vi "Final Project.vi"() -> ()   [LabVIEW 2019]
uses:
  <vilib>/vision/Pattern Matching.llb/IMAQ GM Match Report.ctl
  Control 1.ctl
  <vilib>/MakerHub/LINX/Public/Peripherals/PWM/PWM Set Duty Cycle 1 Chan.vi
  <vilib>/MakerHub/LINX/Public/Peripherals/Digital/Digital Write N Chans.vi
  <vilib>/MakerHub/LINX/Private/Local IO/LinxDigitalWrite.vi
  <vilib>/MakerHub/LINX/Public/Utilities/Check Channel.vi
  <vilib>/MakerHub/LINX/Public/Utilities/Open Serial.vi
  <vilib>/Instr/_visa.llb/VISA Configure Serial Port (Instr).vi
  <vilib>/MakerHub/LINX/Public/Peripherals/PWM/PWM Set Duty Cycle N Chans.vi
  <vilib>/MakerHub/LINX/Private/Utilties/Generate Error.vi
  <vilib>/MakerHub/LINX/LMH-LINX.lvlib
panel:
  in  "Error In":errorcluster
  out "STATE":T1
  out "concatenated string 20":string
  out "concatenated string 19":string
  out "concatenated string 18":string
  out "concatenated string 17":string
  out "concatenated string 16":string
  out "concatenated string 15":string
  out "concatenated string 14":string
  out "concatenated string 13":string
  out "concatenated string 12":string
  out "concatenated string 11":string
  out "concatenated string 10":string
  out "concatenated string 9":string
  out "concatenated string 8":string
  out "concatenated string 7":string
  out "concatenated string 6":string
  out "concatenated string 5":string
  out "concatenated string 4":string
  out "concatenated string 3":string
  out "concatenated string 2":string
  out "concatenated string":string
  out "Calibrated Matches (Pattern Matching 1)":T2[](array[typedef]) {"Correlation Score" format="%.2f"; "Target Template Curve Score" format="%.2f"; "Template Target Curve Score" format="%.2f"; "Bounding Box"."y" format="%.2f"; "Bounding Box"."x" format="%.2f"; "Position"."y" format="%.2f"; "Position"."x" format="%.2f"; "Score" format="%.2f"; "Scale" format="%.2f"; "Angle" format="%.2f"; "Occlusion %" format="%.2f"}
  out "Tab Control":T3(tab)
  in  "Start":bool
  in  "Serial Port":refnum<visa-resource-name>="N/A"
  in  "Duty Cycle (0-1)":dbl(slide) min=0.0 max=1.0 step=5e-05 scale=0.0..1.0
  in  "Values":bool[](array[boolean])
  in  "Start Image Processing":bool
  in  "STOP BUTTON":bool
  in  "OK Button":bool
  out "Jumlah Cawan":i32
  in  "Communicate":bool
  out "Image Out":T4(plugin-control)
  out "1st":cluster{"x":sgl, "y":sgl}
  out "2nd":cluster{"x":sgl, "y":sgl}
  out "3rd":cluster{"x":sgl, "y":sgl}
  out "4th":cluster{"x":sgl, "y":sgl}
  out "5th":cluster{"x":sgl, "y":sgl}
  out "6th":cluster{"x":sgl, "y":sgl}
  out "7th":cluster{"x":sgl, "y":sgl}
  out "8th":cluster{"x":sgl, "y":sgl}
  out "9th":cluster{"x":sgl, "y":sgl}
  out "10th":cluster{"x":sgl, "y":sgl}
  out "11th":cluster{"x":sgl, "y":sgl}
  out "12th":cluster{"x":sgl, "y":sgl}
  out "13th":cluster{"x":sgl, "y":sgl}
  out "14th":cluster{"x":sgl, "y":sgl}
  out "15th":cluster{"x":sgl, "y":sgl}
  out "16th":cluster{"x":sgl, "y":sgl}
  out "17th":cluster{"x":sgl, "y":sgl}
  out "18th":cluster{"x":sgl, "y":sgl}
  out "19th":cluster{"x":sgl, "y":sgl}
  out "20th":cluster{"x":sgl, "y":sgl}
  in  "VISA resource name":refnum<visa-resource-name>="COM1"
  in  "baud rate (9600)":u32=9600
  out "String buat DOBOT":string
  in  "Start Over":bool
  in  "Enum 2":T5(ring)
  in  "SEND!":bool
  out "FEEDBACK":bool
  out "Numeric Control":i32
  out "Response":string
  in  "SENDING DATA":bool
  out "Jumlah Cawan 3":i32
  in  "Termination Character":u8=10 format="%.0x"
  # "SISTEM KENDALI BERBASIS PENGENALAN POLA PADA LENGAN ROBOT \n\"DOBOT\" UNTUK PREPARASI MIKROKAPSUL BRACHYTHERAPY"
  # "Brachytherapy merupakan salah satu bentuk radioterapi dengan menempatkan sumber radiasi sedekat mungkin\natau dimasukkan pada daerah atau jaringan yang rusak akibat kanker. Lengan robot \"DOBOT\" yang didukung \ndengan metode Digital Image Processing yang bertujuan untuk mendeteksi cawan berisi sumber Ir-192 yang akan \ndipindahkan ke dalam mikrokapsul. Aplikasi ini menggunakan metode Digital Image Processing untuk mendeteksi \njumlah dan koordinat posisi cawan dengan menggunakan identifikasi pengenalan pola. Koordinat dan jumlah yang\nterdeteksi akan dikomunikasikan dengan lengan robot menggunakan komunikasi serial."
  # "CREATED AND DEVELOPED BY : DHIYAFATH ANARGYO ORION  - 2021"
  # "CONVEYOR CONTROL"
  # "CONVEYOR SPEED"
  # "MOTOR DIRECTION"
  # "SERIAL PORT"
  # "REVERSE"
  # "FORWARD"
  # "CREATED AND DEVELOPED BY : DHIYAFATH ANARGYO ORION  - 2021"
  # "COORDINATES OF THE CUPS"
  # "AMOUNT OF THE CUPS"
  # "CREATED AND DEVELOPED BY : DHIYAFATH ANARGYO ORION  - 2021"
  # "STRING FOR DOBOT"
  # "SELECT CUP"
  # "AMOUNT OF CUPS"
  # "SERIAL CONFIGURATION"
  # "BAUD RATE"
  # "SERIAL PORT"
  # "RESPONSE"
  # "SENDING DATA"
  # "OFF"
  # "ON"
  # "FEEDBACK"
  # "CREATED AND DEVELOPED BY : DHIYAFATH ANARGYO ORION  - 2021"
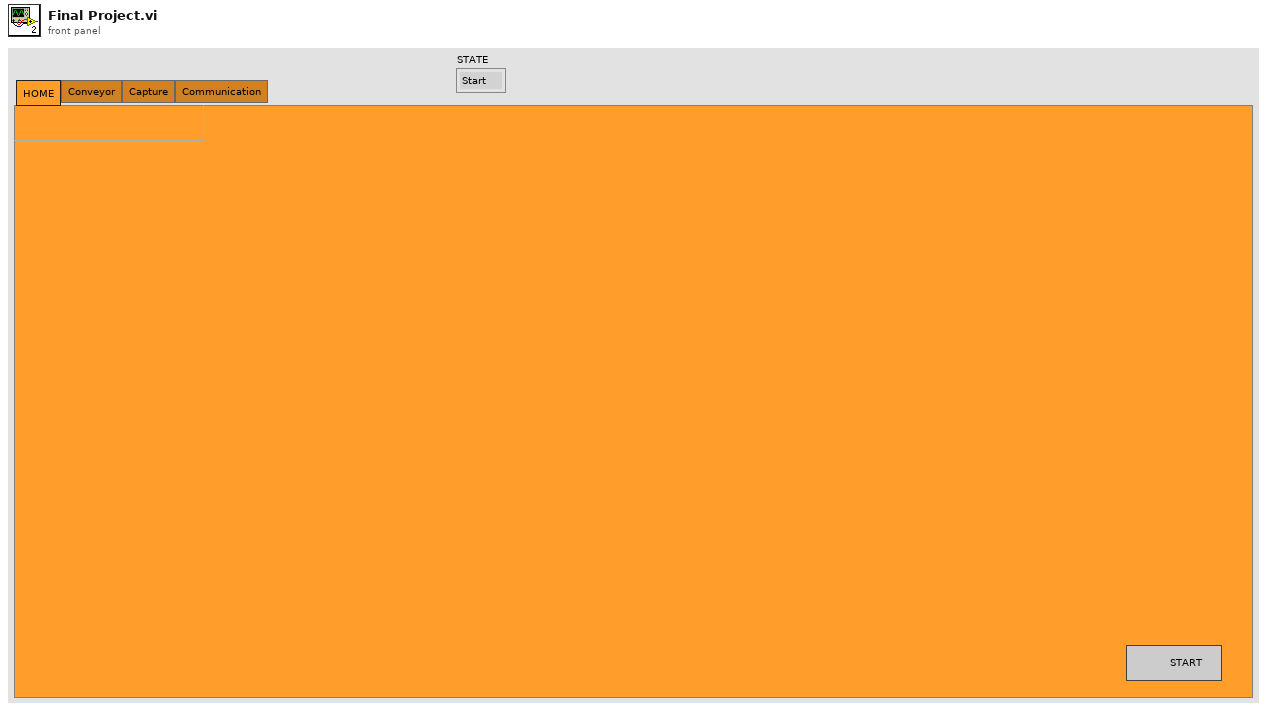
[diagram p1: front panel]
types:
  T1 = typedef "Control 1.ctl" = enum16{"Start", "Conveyor", "Acquire Image", "Process Image", "Sorting", "Sending Data", "Stop"}
  T2 = typedef "IMAQ GM Match Report.ctl" = cluster{"Position":cluster{"x":sgl, "y":sgl}, "Angle":sgl, "Scale":sgl, "Score":sgl, "Bounding Box":cluster{"x":sgl, "y":sgl}[], "Contrast Reversed":bool, "Occlusion %":sgl, "Template Target Curve Score":sgl, "Target Template Curve Score":sgl, "Correlation Score":sgl}
  T3 = enum32{"HOME", "Conveyor", "Capture", "Communication"}
  T4 = typedef "IMAQ Image.ctl" = refnum<image>
  T5 = enum16{"Cawan 1", "Cawan 2", "Cawan 3", "Cawan 4", "Cawan 5", "Cawan 6", "Cawan 7", "Cawan 8", "Cawan 9", "Cawan 10", "Cawan 11", "Cawan 12", "Cawan 13", "Cawan 14", "Cawan 15", "Cawan 16", "Cawan 17", "Cawan 18", "Cawan 19", "Cawan 20"}
  T6 = typedef "LMH-LINX.lvlib/LINX Ref.ctl" = cluster{"IO":T7, "Interface":T8, "LINX Device Config":T9}
  T7 = typedef "LMH-LINX.lvlib/Platform.ctl" = enum16{"Remote", "Local"}
  T8 = typedef "LMH-LINX.lvlib/Interface.ctl" = enum16{"Serial", "TCP"}
  T9 = typedef "LMH-LINX.lvlib/Device.lvlib/LINX Device Config.ctl" = cluster{"Interface":T8, "COM Port":refnum<visa-resource-name>, "TCP Configuration":T10, "Device Family":u8, "Device ID":u8, "Device Name":string, "TCP Ref":refnum<k5>, "Channels":T11}
  T10 = typedef "LMH-LINX.lvlib/Device.lvlib/TCP Config.ctl" = cluster{"IP Address":string, "Port":u16}
  T11 = typedef "LMH-LINX.lvlib/Channels.ctl" = cluster{"DI":u8[], "DO":u8[], "AI":u8[], "AO":u8[], "PWM":u8[], "QE":u8[], "UART":u8[], "I2C 2":u8[], "SPI":u8[], "CAN":u8[], "Servo":u8[], "AI Ref (V)":dbl, "AI Resolution (Bits)":u8, "AO Ref (V)":dbl, "AO Resolution (Bits)":u8}
  T12 = cluster{"[0]":T2, "[1]":T2, "[2]":T2, "[3]":T2, "[4]":T2, "[5]":T2, "[6]":T2, "[7]":T2, "[8]":T2, "[9]":T2, "[10]":T2, "[11]":T2, "[12]":T2, "[13]":T2, "[14]":T2, "[15]":T2, "[16]":T2, "[17]":T2, "[18]":T2, "[19]":T2}
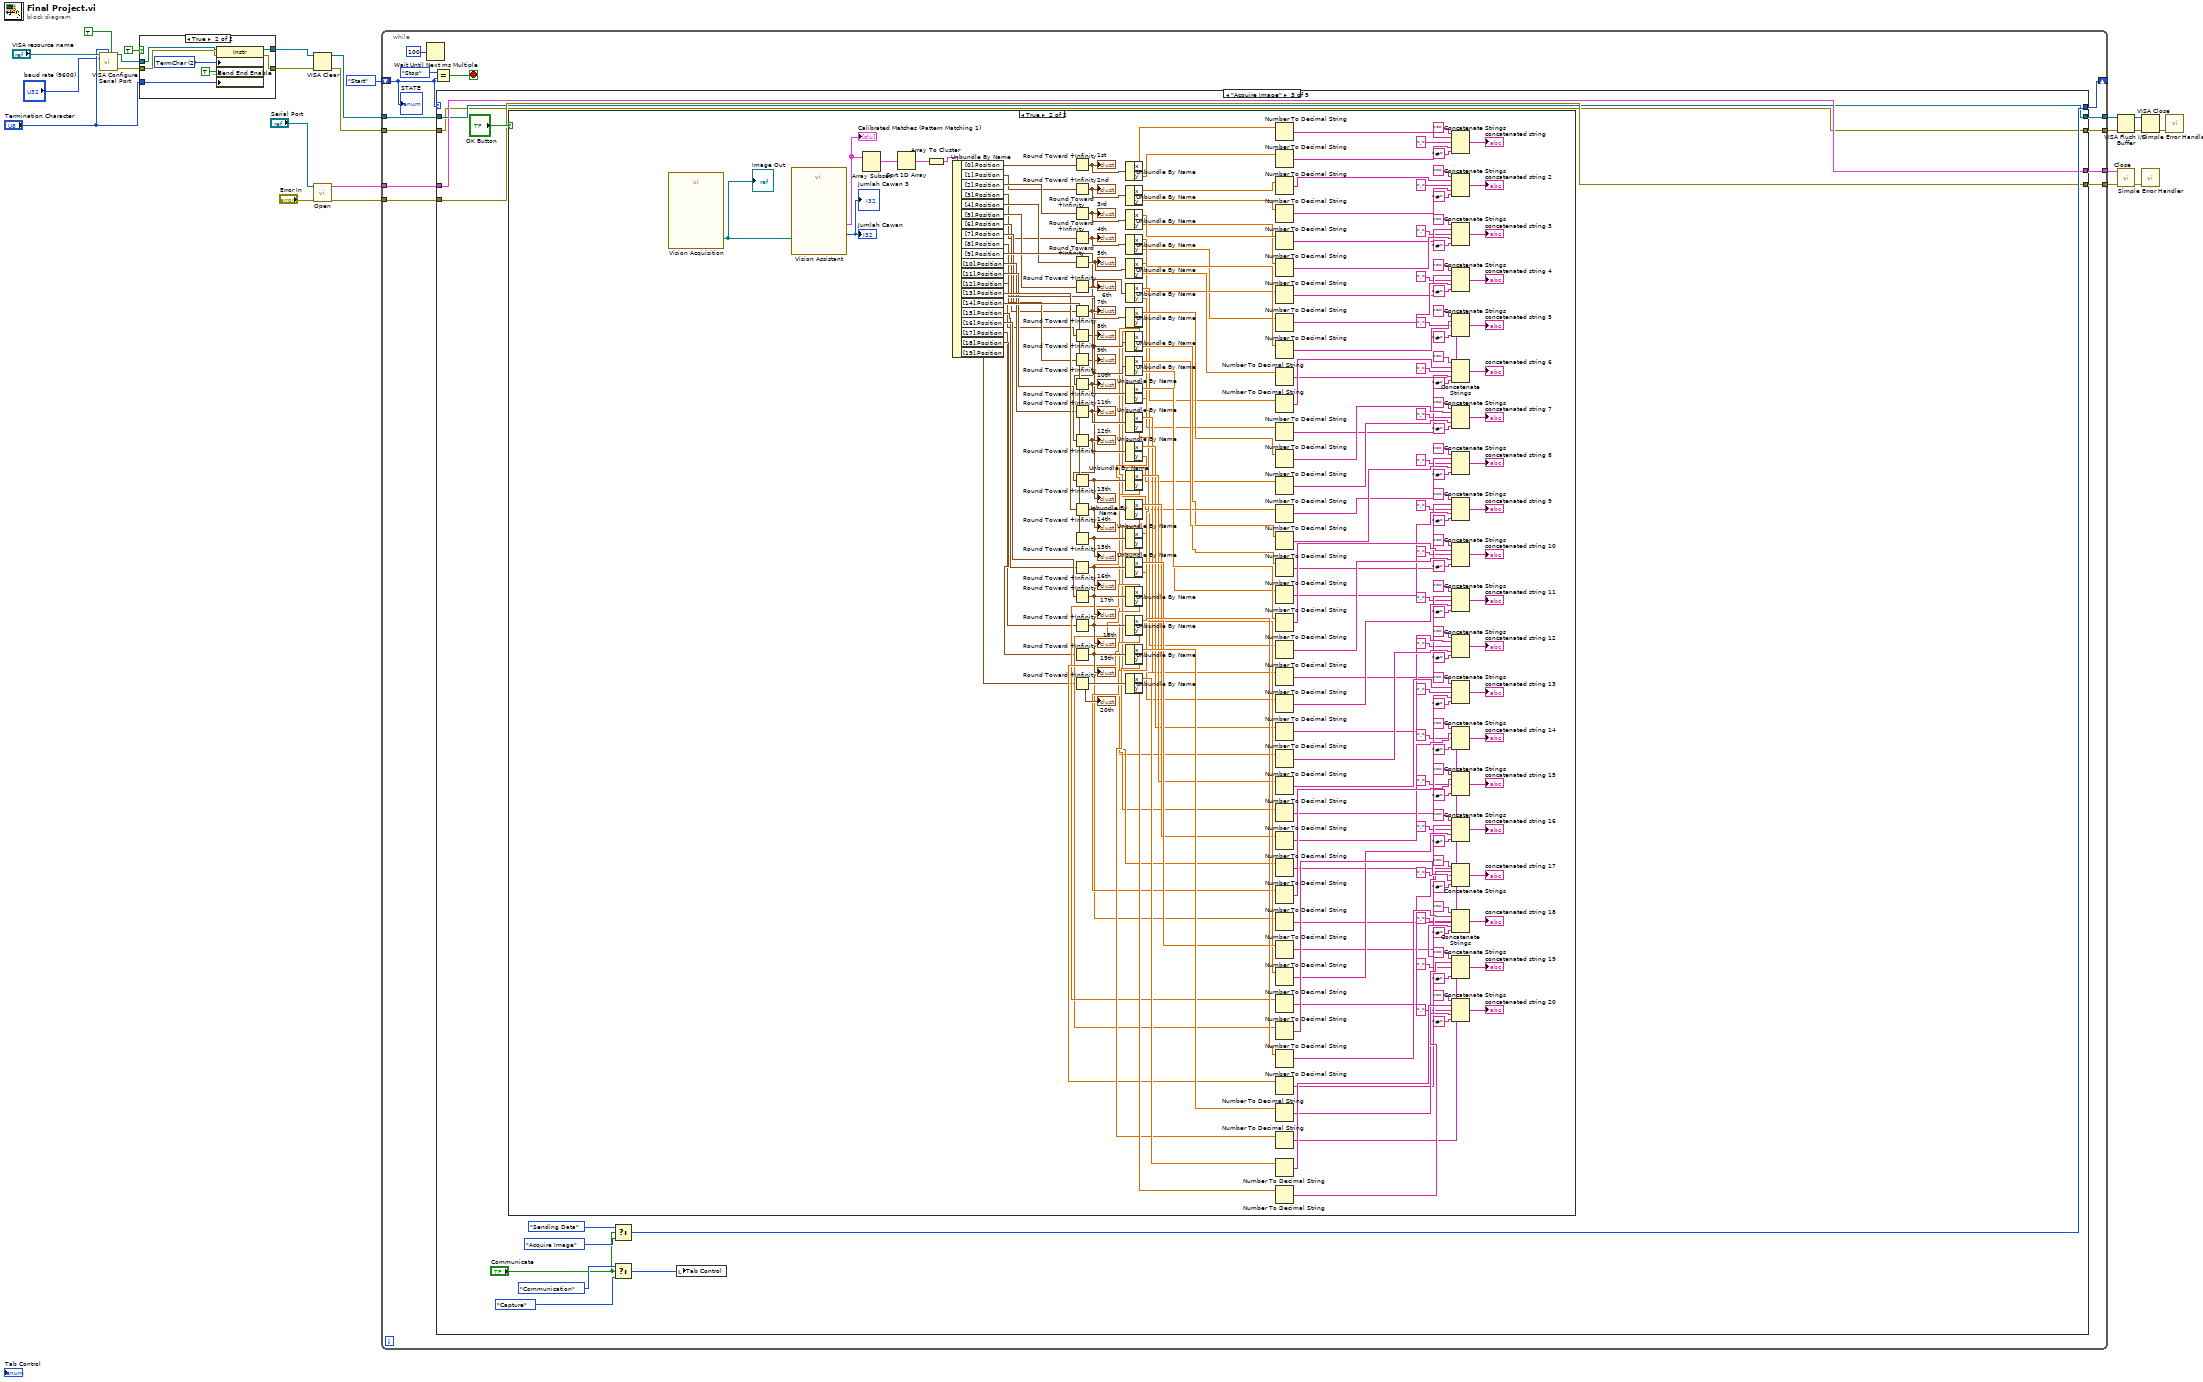
[diagram p0: block diagram]
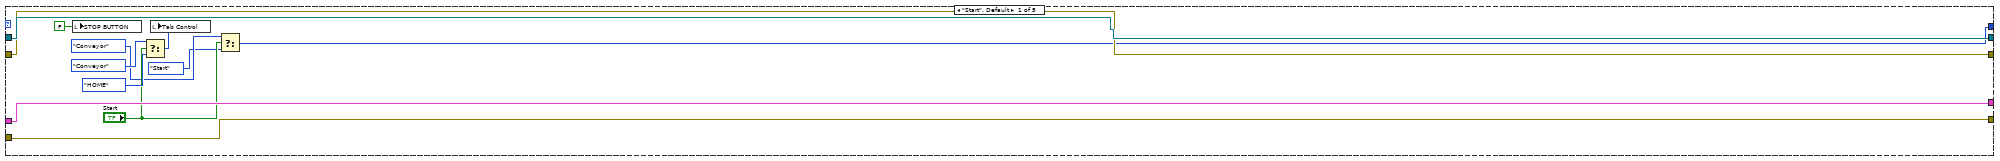
[diagram p3: hidden frame]
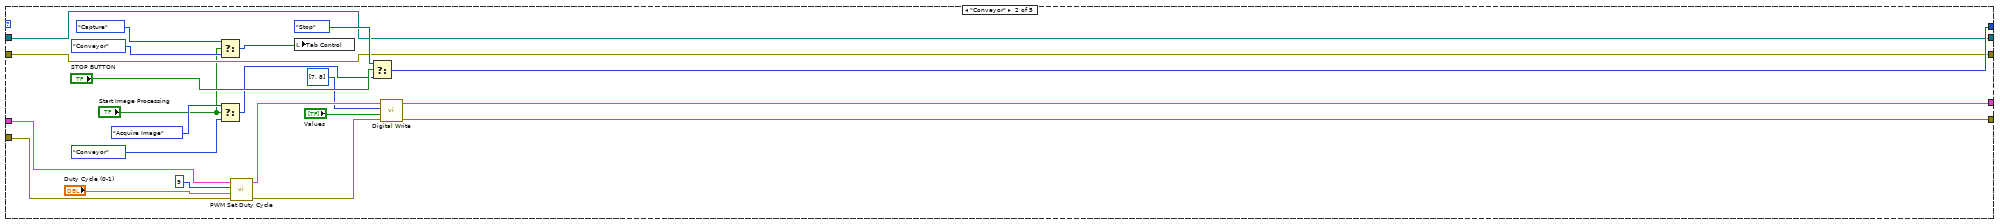
[diagram p4: hidden frame]
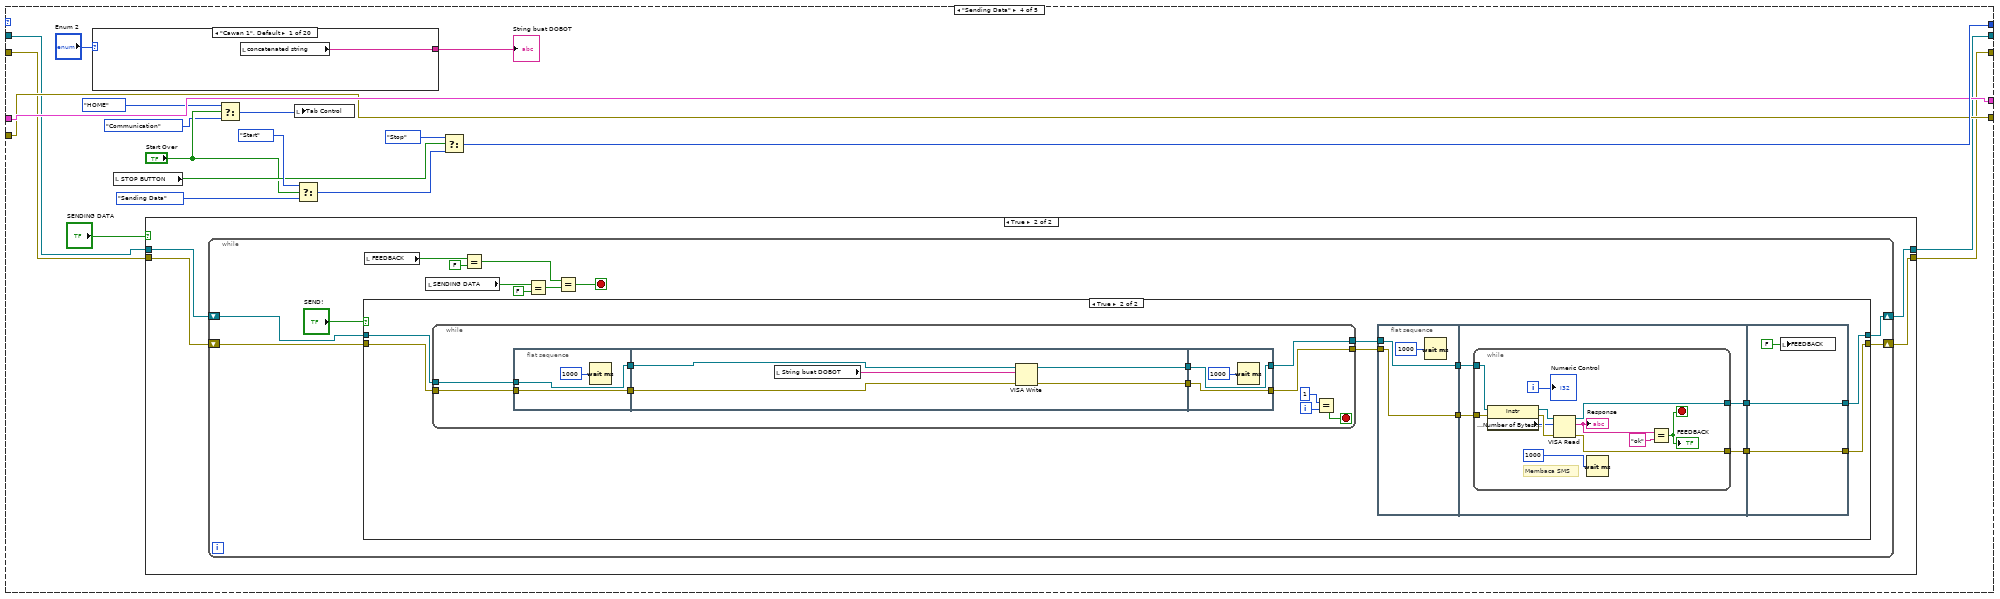
[diagram p6: hidden frame]
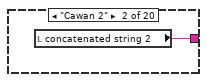
[diagram p9: hidden frame]
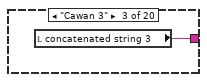
[diagram p10: hidden frame]
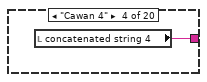
[diagram p11: hidden frame]
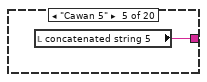
[diagram p12: hidden frame]
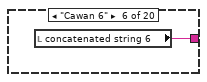
[diagram p13: hidden frame]
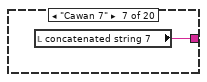
[diagram p14: hidden frame]
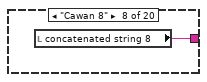
[diagram p15: hidden frame]
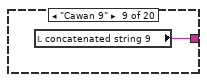
[diagram p16: hidden frame]
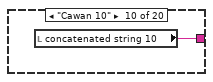
[diagram p17: hidden frame]
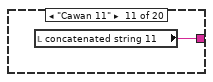
[diagram p18: hidden frame]
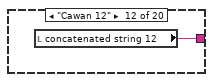
[diagram p19: hidden frame]
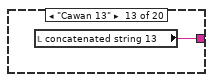
[diagram p20: hidden frame]
diagram:
  n1 = call-poly "VISA Configure Serial Port"("VISA resource name"="VISA resource name", "termination char\n(0xA = '\\n' = LF)"="Termination Character", "Enable Termination\nChar (T)"=TRUE, "baud rate (9600)"="baud rate (9600)") -> ("VISA resource name out"=w9:refnum<visa-resource-name>, "error out"=w8:errorcluster)  [unwired: 6 in, 4 out]
  n2 = case shown="True" TRUE {
    tunnel: w9 -> [w25 w33]
    tunnel: w8 -> [w26 w32]
    tunnel: [w25 w31] -> w7
    tunnel: [w26 w30] -> w6
    tunnel: "Termination Character" -> [_ w28]
    frame False {
    }
    frame True {
      w29 = u16 2 items=["None", "LastBit", "TermChar", "Break"] ("Serial Settings:Serial End Mode for Writes")
      n3 = property class="Instr"(reference=w33, error in=w32, "Serial Settings:End Mode for Writes"=w29, "Message Based Settings:Send End Enable"=TRUE, "Message Based Settings:Termination Character"=w28) -> (reference out=w31:refnum<visa-resource-name>, error out=w30:errorcluster)
    }
  }
  n4 = VISA Clear(VISA resource name=w7, error in (no error)=w6) -> (VISA resource name out=w2:refnum<visa-resource-name>, error out=w1:errorcluster)
  n5 = call-poly <vilib>:"Open.vi"("Error In"="Error In", "Serial Port"="Serial Port") -> ("Error Out"=w19:errorcluster, "LINX Resource"=w20:T6)  [unwired: 7 in, 1 out]
  n6 = while {
    shift-right: [w46] -> _
    shift-left: Control_1."Start" ("STATE") -> [w44]
    tunnel: w20 -> [w41]
    tunnel: w19 -> [w40]
    tunnel: [w39] -> w18
    tunnel: [w38] -> w17
    tunnel: [w37] -> w13
    tunnel: [w36] -> w12
    tunnel: w2 -> [w35]
    tunnel: w1 -> [w34]
    stop <- w45 stop-if-true
    n7 = Wait Until Next ms Multiple(millisecond multiple=u32 100) -> ()  [unwired: 1 out]
    n8 = Equal?(x=Control_1."Stop", y=w44) -> (x = y?=w45:bool)
    n9 = case shown="\"Acquire Image\"" w44 {
      tunnel: [w49 w75 w92 w312 Control_1."Stop" ("x")] -> w46
      tunnel: w41 -> [w57 w68 w88 w311 w414]
      tunnel: w40 -> [w56 w67 w87 w310 w415]
      tunnel: [w57 w65 w88 w311 w414] -> w39
      tunnel: [w56 w66 w87 w310 w415] -> w38
      tunnel: [w55 w64 w86 w307 w413] -> w37
      tunnel: [w54 w63 w85 w306 w412] -> w36
      tunnel: w35 -> [w55 w64 w86 w305 w413]
      tunnel: w34 -> [w54 w63 w85 w304 w412]
      frame "Start", Default {
        n10 = local write "STOP BUTTON"(FALSE ("STOP BUTTON")) -> ()
        n11 = Select(t=T3."Conveyor" ("Tab Control"), s="Start", f=T3."HOME") -> (s? t:f=w47:T3)
        n12 = local write "Tab Control"(w47) -> ()
        n13 = Select(t=Control_1."Conveyor" ("STATE"), s="Start", f=Control_1."Start") -> (s? t:f=w49:T1)
      }
      frame "Conveyor" {
        n14 = Select(t=T3."Capture" ("Tab Control"), s="Start Image Processing", f=T3."Conveyor") -> (s? t:f=w59:T3)
        n15 = Select(t=Control_1."Acquire Image" ("x"), s="Start Image Processing", f=Control_1."Conveyor" ("x")) -> (s? t:f=w77:T1)
        n16 = call-poly <vilib>:"PWM Set Duty Cycle.vi"("Error In"=w67, "Duty Cycle (0-1)"="Duty Cycle (0-1)", "PWM Channel"=u8 9, "LINX Resource"=w68) -> ("Error Out"=w73:errorcluster, "LINX Resource"=w71:T6)  [unwired: 6 in]
        n17 = local write "Tab Control"(w59) -> ()
        n18 = Select(t=Control_1."Stop", s="STOP BUTTON", f=w77) -> (s? t:f=w75:T1)
        n19 = call-poly <vilib>:"Digital Write.vi"("Error In"=w73, "Values"="Values", "DO Channels"=u8[] [7, 8], "LINX Resource"=w71) -> ("Error Out"=w66:errorcluster, "LINX Resource"=w65:T6)  [unwired: 6 in]
      }
      frame "Acquire Image" {
        n20 = case shown="True" "OK Button" {
          frame False {
          }
          frame True {
            n21 = call "Vision Acquisition"() -> ("Image Out"=w298:T4)  [unwired: 26 in, 1 out]
            "Image Out" <- w298
            n22 = call "Vision Assistant"("Image In"=w298) -> ("Calibrated Matches (Pattern Matching 1)"=w94:T2[], "Number of Matches (Pattern Matching 1)"=→"Jumlah Cawan" →"Jumlah Cawan 3":i32)  [unwired: 23 in, 2 out]
            "Calibrated Matches (Pattern Matching 1)" <- w94
            n23 = Array Subset(array=w94) -> (w297:T2[])  [unwired: 2 in]
            n24 = Sort 1D Array(array=w297) -> (sorted array=w155:T2[])
            n25 = Array To Cluster(array=w155) -> (cluster=w156:T12)
            n26 = Unbundle By Name(w156) -> ("[0].Position"=w157:cluster{"x":sgl, "y":sgl}, "[1].Position"=w158:cluster{"x":sgl, "y":sgl}, "[2].Position"=w159:cluster{"x":sgl, "y":sgl}, "[3].Position"=w160:cluster{"x":sgl, "y":sgl}, "[4].Position"=w161:cluster{"x":sgl, "y":sgl}, "[5].Position"=w162:cluster{"x":sgl, "y":sgl}, "[6].Position"=w163:cluster{"x":sgl, "y":sgl}, "[7].Position"=w164:cluster{"x":sgl, "y":sgl}, "[8].Position"=w165:cluster{"x":sgl, "y":sgl}, "[9].Position"=w166:cluster{"x":sgl, "y":sgl}, "[10].Position"=w167:cluster{"x":sgl, "y":sgl}, "[11].Position"=w168:cluster{"x":sgl, "y":sgl}, "[12].Position"=w169:cluster{"x":sgl, "y":sgl}, "[13].Position"=w170:cluster{"x":sgl, "y":sgl}, "[14].Position"=w171:cluster{"x":sgl, "y":sgl}, "[15].Position"=w172:cluster{"x":sgl, "y":sgl}, "[16].Position"=w173:cluster{"x":sgl, "y":sgl}, "[17].Position"=w174:cluster{"x":sgl, "y":sgl}, "[18].Position"=w175:cluster{"x":sgl, "y":sgl}, "[19].Position"=w176:cluster{"x":sgl, "y":sgl})
            n27 = Round Toward +Infinity(x=w157) -> (ceil(x): smallest int >= x=w182:cluster{"x":sgl, "y":sgl})
            "1st" <- w182
            n28 = Round Toward +Infinity(x=w158) -> (ceil(x): smallest int >= x=w277:cluster{"x":sgl, "y":sgl})
            "2nd" <- w277
            n29 = Round Toward +Infinity(x=w159) -> (ceil(x): smallest int >= x=w278:cluster{"x":sgl, "y":sgl})
            "3rd" <- w278
            n30 = Round Toward +Infinity(x=w160) -> (ceil(x): smallest int >= x=w279:cluster{"x":sgl, "y":sgl})
            "4th" <- w279
            n31 = Round Toward +Infinity(x=w161) -> (ceil(x): smallest int >= x=w280:cluster{"x":sgl, "y":sgl})
            "5th" <- w280
            n32 = Round Toward +Infinity(x=w162) -> (ceil(x): smallest int >= x=w281:cluster{"x":sgl, "y":sgl})
            "6th" <- w281
            n33 = Round Toward +Infinity(x=w163) -> (ceil(x): smallest int >= x=w282:cluster{"x":sgl, "y":sgl})
            "7th" <- w282
            n34 = Round Toward +Infinity(x=w164) -> (ceil(x): smallest int >= x=w283:cluster{"x":sgl, "y":sgl})
            "8th" <- w283
            n35 = Round Toward +Infinity(x=w165) -> (ceil(x): smallest int >= x=w285:cluster{"x":sgl, "y":sgl})
            "9th" <- w285
            n36 = Round Toward +Infinity(x=w166) -> (ceil(x): smallest int >= x=w286:cluster{"x":sgl, "y":sgl})
            "10th" <- w286
            n37 = Round Toward +Infinity(x=w167) -> (ceil(x): smallest int >= x=w287:cluster{"x":sgl, "y":sgl})
            "11th" <- w287
            n38 = Round Toward +Infinity(x=w168) -> (ceil(x): smallest int >= x=w288:cluster{"x":sgl, "y":sgl})
            "12th" <- w288
            n39 = Round Toward +Infinity(x=w169) -> (ceil(x): smallest int >= x=w289:cluster{"x":sgl, "y":sgl})
            "13th" <- w289
            n40 = Round Toward +Infinity(x=w170) -> (ceil(x): smallest int >= x=w290:cluster{"x":sgl, "y":sgl})
            "14th" <- w290
            n41 = Round Toward +Infinity(x=w171) -> (ceil(x): smallest int >= x=w291:cluster{"x":sgl, "y":sgl})
            "15th" <- w291
            n42 = Round Toward +Infinity(x=w172) -> (ceil(x): smallest int >= x=w296:cluster{"x":sgl, "y":sgl})
            "16th" <- w296
            n43 = Round Toward +Infinity(x=w173) -> (ceil(x): smallest int >= x=w292:cluster{"x":sgl, "y":sgl})
            "17th" <- w292
            n44 = Round Toward +Infinity(x=w174) -> (ceil(x): smallest int >= x=w295:cluster{"x":sgl, "y":sgl})
            "18th" <- w295
            n45 = Round Toward +Infinity(x=w175) -> (ceil(x): smallest int >= x=w293:cluster{"x":sgl, "y":sgl})
            "19th" <- w293
            n46 = Round Toward +Infinity(x=w176) -> (ceil(x): smallest int >= x=w294:cluster{"x":sgl, "y":sgl})
            "20th" <- w294
            n47 = Unbundle By Name(w182) -> ("x"=w181:sgl, "y"=w177:sgl)
            n48 = Unbundle By Name(w277) -> ("x"=w186:sgl, "y"=w183:sgl)
            n49 = Unbundle By Name(w278) -> ("x"=w191:sgl, "y"=w187:sgl)
            n50 = Unbundle By Name(w279) -> ("x"=w196:sgl, "y"=w192:sgl)
            n51 = Unbundle By Name(w280) -> ("x"=w201:sgl, "y"=w197:sgl)
            n52 = Unbundle By Name(w281) -> ("x"=w206:sgl, "y"=w202:sgl)
            n53 = Unbundle By Name(w282) -> ("x"=w211:sgl, "y"=w207:sgl)
            n54 = Unbundle By Name(w283) -> ("x"=w216:sgl, "y"=w212:sgl)
            n55 = Unbundle By Name(w285) -> ("x"=w221:sgl, "y"=w217:sgl)
            n56 = Unbundle By Name(w286) -> ("x"=w226:sgl, "y"=w222:sgl)
            n57 = Unbundle By Name(w287) -> ("x"=w231:sgl, "y"=w227:sgl)
            n58 = Unbundle By Name(w288) -> ("x"=w236:sgl, "y"=w232:sgl)
            n59 = Unbundle By Name(w289) -> ("x"=w237:sgl, "y"=w241:sgl)
            n60 = Unbundle By Name(w290) -> ("x"=w246:sgl, "y"=w242:sgl)
            n61 = Unbundle By Name(w291) -> ("x"=w251:sgl, "y"=w247:sgl)
            n62 = Unbundle By Name(w296) -> ("x"=w256:sgl, "y"=w252:sgl)
            n63 = Unbundle By Name(w292) -> ("x"=w261:sgl, "y"=w257:sgl)
            n64 = Unbundle By Name(w295) -> ("x"=w266:sgl, "y"=w262:sgl)
            n65 = Unbundle By Name(w293) -> ("x"=w271:sgl, "y"=w267:sgl)
            n66 = Unbundle By Name(w294) -> ("x"=w276:sgl, "y"=w272:sgl)
            n67 = Number To Decimal String(number=w181) -> (decimal integer string=w179:string)  [unwired: 1 in]
            n68 = Number To Decimal String(number=w177) -> (decimal integer string=w180:string)  [unwired: 1 in]
            n69 = Number To Decimal String(number=w186) -> (decimal integer string=w184:string)  [unwired: 1 in]
            n70 = Number To Decimal String(number=w183) -> (decimal integer string=w185:string)  [unwired: 1 in]
            n71 = Number To Decimal String(number=w191) -> (decimal integer string=w189:string)  [unwired: 1 in]
            n72 = Number To Decimal String(number=w187) -> (decimal integer string=w190:string)  [unwired: 1 in]
            n73 = Number To Decimal String(number=w196) -> (decimal integer string=w194:string)  [unwired: 1 in]
            n74 = Number To Decimal String(number=w192) -> (decimal integer string=w195:string)  [unwired: 1 in]
            n75 = Number To Decimal String(number=w201) -> (decimal integer string=w199:string)  [unwired: 1 in]
            n76 = Number To Decimal String(number=w197) -> (decimal integer string=w200:string)  [unwired: 1 in]
            n77 = Number To Decimal String(number=w206) -> (decimal integer string=w204:string)  [unwired: 1 in]
            n78 = Number To Decimal String(number=w202) -> (decimal integer string=w205:string)  [unwired: 1 in]
            n79 = Number To Decimal String(number=w211) -> (decimal integer string=w209:string)  [unwired: 1 in]
            n80 = Number To Decimal String(number=w207) -> (decimal integer string=w210:string)  [unwired: 1 in]
            n81 = Number To Decimal String(number=w216) -> (decimal integer string=w214:string)  [unwired: 1 in]
            n82 = Number To Decimal String(number=w212) -> (decimal integer string=w215:string)  [unwired: 1 in]
            n83 = Number To Decimal String(number=w221) -> (decimal integer string=w219:string)  [unwired: 1 in]
            n84 = Number To Decimal String(number=w217) -> (decimal integer string=w220:string)  [unwired: 1 in]
            n85 = Number To Decimal String(number=w226) -> (decimal integer string=w224:string)  [unwired: 1 in]
            n86 = Number To Decimal String(number=w222) -> (decimal integer string=w225:string)  [unwired: 1 in]
            n87 = Number To Decimal String(number=w231) -> (decimal integer string=w229:string)  [unwired: 1 in]
            n88 = Number To Decimal String(number=w227) -> (decimal integer string=w230:string)  [unwired: 1 in]
            n89 = Number To Decimal String(number=w236) -> (decimal integer string=w234:string)  [unwired: 1 in]
            n90 = Number To Decimal String(number=w232) -> (decimal integer string=w235:string)  [unwired: 1 in]
            n91 = Number To Decimal String(number=w237) -> (decimal integer string=w239:string)  [unwired: 1 in]
            n92 = Number To Decimal String(number=w241) -> (decimal integer string=w238:string)  [unwired: 1 in]
            n93 = Number To Decimal String(number=w246) -> (decimal integer string=w244:string)  [unwired: 1 in]
            n94 = Number To Decimal String(number=w242) -> (decimal integer string=w245:string)  [unwired: 1 in]
            n95 = Number To Decimal String(number=w251) -> (decimal integer string=w249:string)  [unwired: 1 in]
            n96 = Number To Decimal String(number=w247) -> (decimal integer string=w250:string)  [unwired: 1 in]
            n97 = Number To Decimal String(number=w256) -> (decimal integer string=w254:string)  [unwired: 1 in]
            n98 = Number To Decimal String(number=w252) -> (decimal integer string=w255:string)  [unwired: 1 in]
            n99 = Number To Decimal String(number=w261) -> (decimal integer string=w259:string)  [unwired: 1 in]
            n100 = Number To Decimal String(number=w257) -> (decimal integer string=w260:string)  [unwired: 1 in]
            n101 = Number To Decimal String(number=w266) -> (decimal integer string=w264:string)  [unwired: 1 in]
            n102 = Number To Decimal String(number=w262) -> (decimal integer string=w265:string)  [unwired: 1 in]
            n103 = Number To Decimal String(number=w271) -> (decimal integer string=w269:string)  [unwired: 1 in]
            n104 = Number To Decimal String(number=w267) -> (decimal integer string=w270:string)  [unwired: 1 in]
            n105 = Number To Decimal String(number=w276) -> (decimal integer string=w274:string)  [unwired: 1 in]
            n106 = Number To Decimal String(number=w272) -> (decimal integer string=w275:string)  [unwired: 1 in]
            n107 = Concatenate Strings("*" ("string"), w179, "," ("string"), w180, "#" ("string")) -> (→"concatenated string":string)
            n108 = Concatenate Strings("*" ("string"), w184, "," ("string"), w185, "#" ("string")) -> (→"concatenated string 2":string)
            n109 = Concatenate Strings("*" ("string"), w189, "," ("string"), w190, "#" ("string")) -> (→"concatenated string 3":string)
            n110 = Concatenate Strings("*" ("string"), w194, "," ("string"), w195, "#" ("string")) -> (→"concatenated string 4":string)
            n111 = Concatenate Strings("*" ("string"), w199, "," ("string"), w200, "#" ("string")) -> (→"concatenated string 5":string)
            n112 = Concatenate Strings("*" ("string"), w204, "," ("string"), w205, "#" ("string")) -> (→"concatenated string 6":string)
            n113 = Concatenate Strings("*" ("string"), w209, "," ("string"), w210, "#" ("string")) -> (→"concatenated string 7":string)
            n114 = Concatenate Strings("*" ("string"), w214, "," ("string"), w215, "#" ("string")) -> (→"concatenated string 8":string)
            n115 = Concatenate Strings("*" ("string"), w219, "," ("string"), w220, "#" ("string")) -> (→"concatenated string 9":string)
            n116 = Concatenate Strings("*" ("string"), w224, "," ("string"), w225, "#" ("string")) -> (→"concatenated string 10":string)
            n117 = Concatenate Strings("*" ("string"), w229, "," ("string"), w230, "#" ("string")) -> (→"concatenated string 11":string)
            n118 = Concatenate Strings("*" ("string"), w234, "," ("string"), w235, "#" ("string")) -> (→"concatenated string 12":string)
            n119 = Concatenate Strings("*" ("string"), w239, "," ("string"), w238, "#" ("string")) -> (→"concatenated string 13":string)
            n120 = Concatenate Strings("*" ("string"), w244, "," ("string"), w245, "#" ("string")) -> (→"concatenated string 14":string)
            n121 = Concatenate Strings("*" ("string"), w249, "," ("string"), w250, "#" ("string")) -> (→"concatenated string 15":string)
            n122 = Concatenate Strings("*" ("string"), w254, "," ("string"), w255, "#" ("string")) -> (→"concatenated string 16":string)
            n123 = Concatenate Strings("*" ("string"), w259, "," ("string"), w260, "#" ("string")) -> (→"concatenated string 17":string)
            n124 = Concatenate Strings("*" ("string"), w264, "," ("string"), w265, "#" ("string")) -> (→"concatenated string 18":string)
            n125 = Concatenate Strings("*" ("string"), w269, "," ("string"), w270, "#" ("string")) -> (→"concatenated string 19":string)
            n126 = Concatenate Strings("*" ("string"), w274, "," ("string"), w275, "#" ("string")) -> (→"concatenated string 20":string)
          }
        }
        n127 = Select(t=Control_1."Sending Data" ("x"), s="Communicate", f=Control_1."Acquire Image" ("x")) -> (s? t:f=w92:T1)
        n128 = Select(t=T3."Communication" ("Tab Control"), s="Communicate", f=T3."Capture") -> (s? t:f=w81:T3)
        n129 = local write "Tab Control"(w81) -> ()
      }
      frame "Sending Data" {
        n130 = case shown="\"Cawan 1\", Default" "Enum 2" {
          tunnel: [w392 w393 w394 w395 w396 w397 w398 w399 w400 w401 w402 w403 w404 w405 w406 w407 w408 w409 w410 w411] -> w308
          frame "Cawan 1", Default {
            n131 = local read "concatenated string"() -> (w392:string)
          }
          frame "Cawan 2" {
            n132 = local read "concatenated string 2"() -> (w393:string)
          }
          frame "Cawan 3" {
            n133 = local read "concatenated string 3"() -> (w394:string)
          }
          frame "Cawan 4" {
            n134 = local read "concatenated string 4"() -> (w395:string)
          }
          frame "Cawan 5" {
            n135 = local read "concatenated string 5"() -> (w396:string)
          }
          frame "Cawan 6" {
            n136 = local read "concatenated string 6"() -> (w397:string)
          }
          frame "Cawan 7" {
            n137 = local read "concatenated string 7"() -> (w398:string)
          }
          frame "Cawan 8" {
            n138 = local read "concatenated string 8"() -> (w399:string)
          }
          frame "Cawan 9" {
            n139 = local read "concatenated string 9"() -> (w400:string)
          }
          frame "Cawan 10" {
            n140 = local read "concatenated string 10"() -> (w401:string)
          }
          frame "Cawan 11" {
            n141 = local read "concatenated string 11"() -> (w402:string)
          }
          frame "Cawan 12" {
            n142 = local read "concatenated string 12"() -> (w403:string)
          }
          frame "Cawan 13" {
            n143 = local read "concatenated string 13"() -> (w404:string)
          }
          frame "Cawan 14" {
            n144 = local read "concatenated string 14"() -> (w405:string)
          }
          frame "Cawan 15" {
            n145 = local read "concatenated string 15"() -> (w406:string)
          }
          frame "Cawan 16" {
            n146 = local read "concatenated string 16"() -> (w407:string)
          }
          frame "Cawan 17" {
            n147 = local read "concatenated string 17"() -> (w408:string)
          }
          frame "Cawan 18" {
            n148 = local read "concatenated string 18"() -> (w409:string)
          }
          frame "Cawan 19" {
            n149 = local read "concatenated string 19"() -> (w410:string)
          }
          frame "Cawan 20" {
            n150 = local read "concatenated string 20"() -> (w411:string)
          }
        }
        "String buat DOBOT" <- w308
        n151 = local read "STOP BUTTON"() -> (w314:bool)
        n152 = case shown="True" "SENDING DATA" {
          tunnel: [w319 w323] -> w307
          tunnel: [w318 w322] -> w306
          tunnel: w305 -> [w319 w321]
          tunnel: w304 -> [w318 w320]
          frame False {
          }
          frame True {
            n153 = while {
              shift-right: [w334] -> w322
              shift-left: w320 -> [w333]
              shift-right: [w335] -> w323
              shift-left: w321 -> [w332]
              stop <- w325 stop-if-true
              n154 = case shown="True" "SEND!" {
                tunnel: [w337 w345] -> w335
                tunnel: [w336 w344] -> w334
                tunnel: w333 -> [w336 w340]
                tunnel: w332 -> [w337 w341]
                frame False {
                }
                frame True {
                  n155 = while {
                    tunnel: w341 -> [w356]
                    tunnel: [w354] -> w343
                    tunnel: w340 -> [w355]
                    tunnel: [w353] -> w342
                    i -> [w352]
                    stop <- w350 stop-if-true
                    n156 = flat-sequence {
                      tunnel: w355 -> [w360]
                      tunnel: w356 -> [w361]
                      tunnel: [w361] -> w349
                      tunnel: [w360] -> w348
                      tunnel: [w366] -> w358
                      tunnel: [w365] -> w357
                      tunnel: w349 -> [w364]
                      tunnel: w348 -> [w363]
                      tunnel: w358 -> [w368]
                      tunnel: w357 -> [w367]
                      tunnel: [w368] -> w354
                      tunnel: [w367] -> w353
                      frame #0 {
                        n157 = Wait (ms)(milliseconds to wait=u32 1000) -> ()  [unwired: 1 out]
                      }
                      frame #1 {
                        n158 = local read "String buat DOBOT"() -> (w362:string)
                        n159 = VISA Write(VISA resource name=w364, write buffer=w362, error in (no error)=w363) -> (VISA resource name out=w366:refnum<visa-resource-name>, error out=w365:errorcluster)  [unwired: 1 out]
                      }
                      frame #2 {
                        n160 = Wait (ms)(milliseconds to wait=u32 1000) -> ()  [unwired: 1 out]
                      }
                    }
                    n161 = Equal?(x=1, y=w352) -> (x = y?=w350:bool)
                  }
                  n162 = flat-sequence {
                    tunnel: [w371] -> w347
                    tunnel: w342 -> [w371]
                    tunnel: w343 -> [w370]
                    tunnel: [w370] -> w346
                    tunnel: w347 -> [w376]
                    tunnel: w346 -> [w375]
                    tunnel: [w374] -> w339
                    tunnel: [w373] -> w338
                    tunnel: [w390] -> w344
                    tunnel: [w391] -> w345
                    tunnel: w339 -> [w391]
                    tunnel: w338 -> [w390]
                    frame #0 {
                      n163 = Wait (ms)(milliseconds to wait=u32 1000) -> ()  [unwired: 1 out]
                    }
                    frame #1 {
                      n164 = while {
                        tunnel: [w386] -> w374
                        tunnel: [w385] -> w373
                        tunnel: w376 -> [w383]
                        tunnel: w375 -> [w382]
                        i -> [w378]
                        stop <- w377 stop-if-true
                        # "Membaca SMS"
                        n165 = property class="Instr"(reference=w382, error in=w383) -> (reference out=w388:refnum<visa-resource-name>, error out=w387:errorcluster, "Serial Settings:Number of Bytes at Serial Port"=w384:u32)
                        n166 = VISA Read(VISA resource name=w388, byte count=w384, error in (no error)=w387) -> (VISA resource name out=w386:refnum<visa-resource-name>, read buffer=w380:string, error out=w385:errorcluster)  [unwired: 1 out]
                        "Response" <- w380
                        n167 = Wait (ms)(milliseconds to wait=u32 1000) -> ()  [unwired: 1 out]
                        n168 = Equal?(x=w380, y="ok") -> (x = y?=w377:bool)
                        "FEEDBACK" <- w377
                        "Numeric Control" <- w378
                      }
                    }
                    frame #2 {
                      n169 = local write "FEEDBACK"(FALSE ("x = y?")) -> ()
                    }
                  }
                }
              }
              n170 = local read "FEEDBACK"() -> (w330:bool)
              n171 = local read "SENDING DATA"() -> (w328:bool)
              n172 = Equal?(x=w330, y=FALSE) -> (x = y?=w327:bool)
              n173 = Equal?(x=w328, y=FALSE) -> (x = y?=w326:bool)
              n174 = Equal?(x=w327, y=w326) -> (x = y?=w325:bool)
            }
          }
        }
        n175 = Select(t=T3."HOME" ("Tab Control"), s="Start Over", f=T3."Communication") -> (s? t:f=w300:T3)
        n176 = local write "Tab Control"(w300) -> ()
        n177 = Select(t=Control_1."Start" ("x"), s="Start Over", f=Control_1."Sending Data" ("x")) -> (s? t:f=w315:T1)
        n178 = Select(t=Control_1."Stop", s=w314, f=w315) -> (s? t:f=w312:T1)
      }
      frame "Stop" {
      }
    }
    "STATE" <- w44
  }
  n179 = VISA Flush I/O Buffer(VISA resource name=w13, error in (no error)=w12) -> (VISA resource name out=w15:refnum<visa-resource-name>, error out=w16:errorcluster)  [unwired: 1 in]
  n180 = call <vilib>:"Close.vi"("Error In"=w17, "LINX Resource"=w18) -> ("Error Out"=w23:errorcluster)  [unwired: 9 in]
  n181 = VISA Close(VISA resource name=w15, error in (no error)=w16) -> (error out=w14:errorcluster)
  n182 = call <vilib>:"Simple Error Handler.vi"("error in (no error)"=w23) -> ()  [unwired: 4 in, 5 out]
  n183 = call <vilib>:"Simple Error Handler.vi"("error in (no error)"=w14) -> ()  [unwired: 4 in, 5 out]
